vi "GD_GesamtKonz_back_calc.vi"(6 "ohne Einheiten":bool, 7 "Gesamtkonzentration":dbl, 8 "Einheiten":string[](array[string]), 9 "Konzentration der Komponenten":dbl[](array[numeric]), 10 "Stufen":string[](array[string]), 11 "Punkte (Eingang)":string[](array[string])) -> (2 "Stufen Array":string[][](array[string]), 3 "Stufentabellen (Ausgang)":string[][][](array[string]))   [LabVIEW 2020, in "Linearisierung v2.lvlib" / "Gasteiler.lvlib"]
uses:
  Gasteiler.lvlib
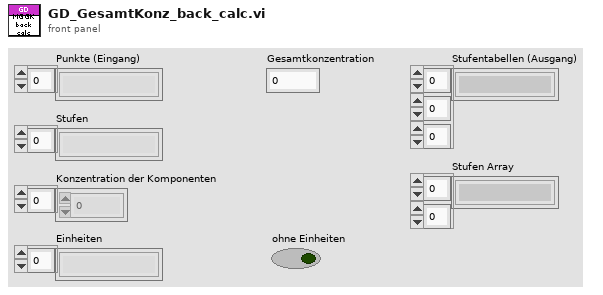
[diagram p1: front panel]
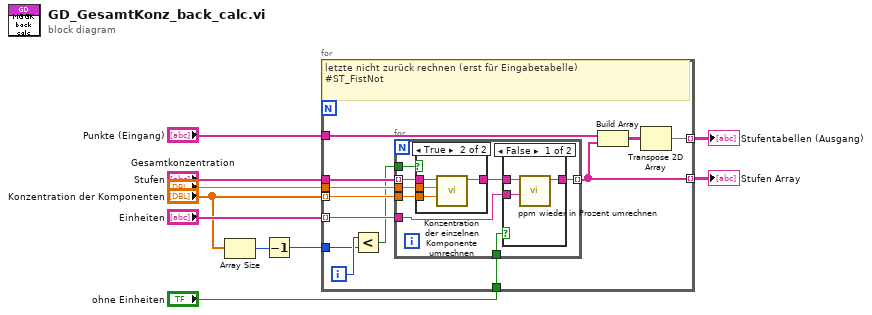
[diagram p0: block diagram]
diagram:
  n1 = Array Size(array="Konzentration der Komponenten") -> (size(s)=w4:i32)
  n2 = Decrement(x=w4) -> (x-1=w3:i32)
  n3 = for {
    tunnel: "Konzentration der Komponenten" -> [w22] mode=indexing
    tunnel: "Einheiten" -> [w21] mode=indexing
    tunnel: "Stufen" -> [w20]
    tunnel: "Gesamtkonzentration" -> [w19]
    tunnel: "Punkte (Eingang)" -> [w17]
    tunnel: [w16] -> w10 mode=indexing
    tunnel: w3 -> [w14]
    tunnel: "ohne Einheiten" -> [w12]
    tunnel: [w11] -> w1 mode=indexing
    i -> [w15]
    # "letzte nicht zurück rechnen (erst für Eingabetabelle)\n#ST_FistNot"
    n4 = Less?(x=w15, y=w14) -> (x < y?=w13:bool)
    n5 = for {
      tunnel: w22 -> [w28]
      tunnel: w21 -> [w27]
      tunnel: w20 -> [w29] mode=indexing
      tunnel: w19 -> [w26]
      tunnel: [w25] -> w11 mode=indexing
      tunnel: w13 -> [w24]
      tunnel: w12 -> [w23]
      n6 = case shown="True" w24 {
        tunnel: [w35 w39] -> w30
        tunnel: w29 -> [w35 w38]
        tunnel: w28 -> [_ w37]
        tunnel: w26 -> [_ w36]
        frame False {
        }
        frame True {
          n7 = call "Konzentration der einzelnen Komponente umrechnen.vi"("Teilkonzentration"=w37, "Gesamtkonzentration"=w36, "Werteingang"=w38) -> ("Wertausgang"=w39:string)  [unwired: 8 in]
        }
      }
      n8 = case shown="False" w23 {
        tunnel: w30 -> [w33 w34]
        tunnel: w27 -> [w32 _]
        tunnel: [w31 w34] -> w25
        frame False {
          n9 = call "ppm wieder in Prozent umrechnen.vi"("Einheit"=w32, "Werteingang"=w33) -> ("Wertausgang"=w31:string)  [unwired: 9 in]
        }
        frame True {
        }
      }
    }
    n10 = Build Array(w17, w11) -> (w18:string[][])
    n11 = Transpose 2D Array(2D array=w18) -> (transposed array=w16:string[][])
  }
  "Stufentabellen (Ausgang)" <- w10
  "Stufen Array" <- w1
